vi "ReversedEngineering AttributesTypeToString.vi"(1 "AttributeDataType":T1, 2 "name":string) -> (15 "string":string)   [LabVIEW 2016]
uses:
  <resource>/Framework/Providers/Open_GDS/ClassProviders/Common/CommonVIs/CommonVIs_AttributeDataType.ctl
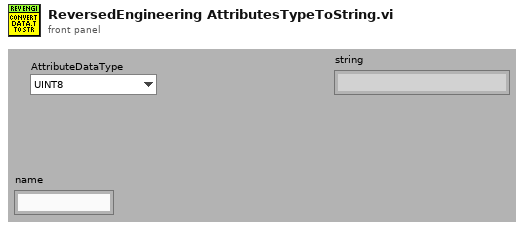
[diagram p1: front panel]
types:
  T1 = typedef "CommonVIs_AttributeDataType.ctl" = enum16{"UINT8", "INT8", "UINT16", "INT16", "UINT32", "INT32", "UINT64", "INT64", "SGL", "DBL", "EXT", "CSG", "CDB", "CXT", "TimeStamp", "STRING", "PATH", "BOOL", "ENUM", "RefNum", "VIRefNum", "LabVIEW Class", "Cluster", "Variant", "TypeDef", "Waveform", "LabVIEW Object", "Other", "void"}
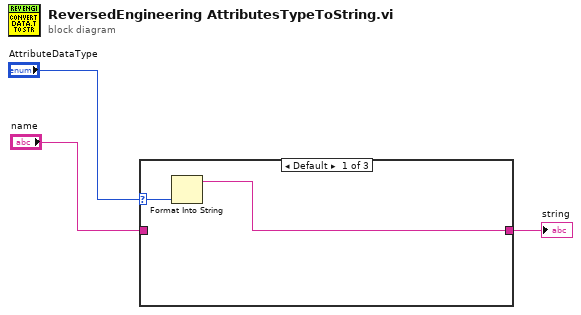
[diagram p0: block diagram]
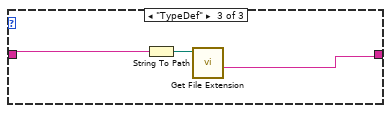
[diagram p3: hidden frame]
diagram:
  n1 = case shown="Default" "AttributeDataType" {
    selector: "AttributeDataType" -> [w5 _ _]
    tunnel: "name" -> [_ w6 w9]
    tunnel: [w4 w6 w7] -> w1
    frame Default {
      n2 = Format Into String(w5) -> (resulting string=w4:string)  [unwired: 3 in, 1 out]
    }
    frame "LabVIEW Class" {
    }
    frame "TypeDef" {
      n3 = String To Path(string=w9) -> (path=w8:path)
      n4 = call <vilib>:"Get File Extension.vi"("file"=w8) -> ("filename without extension"=w7:string)  [unwired: 1 in, 9 out]
    }
  }
  "string" <- w1
